vi "Chronos TDMS File Viewer Add Plot.vi"(4 "Data Units":string, 6 "Group":string, 8 "Times":dbl[](array[numeric]), 9 "Data":dbl[](array[numeric]), 10 "Name":string, 11 "Limit Plot Map":T1) -> (3 "Plot Map out":T1)   [LabVIEW 2021]
uses:
  GUI/Chronos cluster Map Limit Plots.ctl
  typedefs/Chronos cluster Plot Data and Limits.ctl
  cluster CC Channel from TDMS.ctl
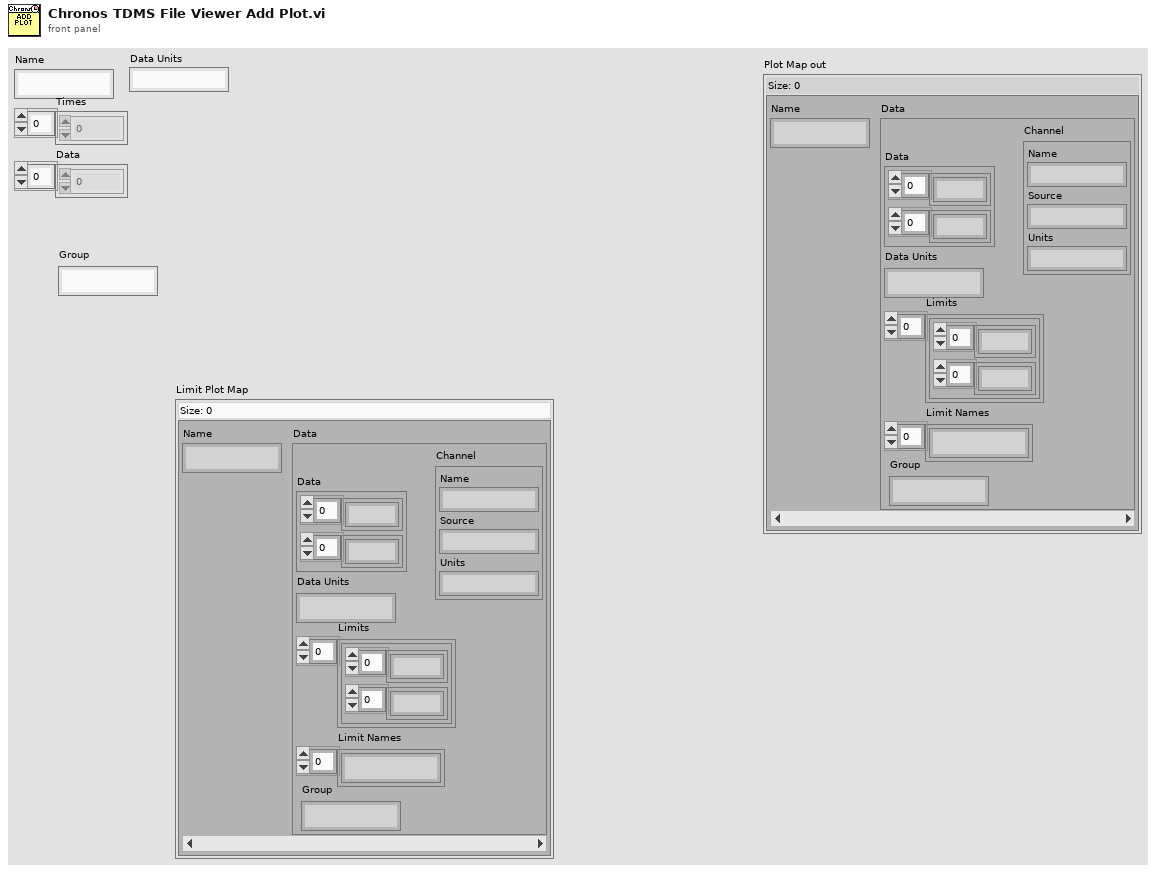
[diagram p1: front panel]
types:
  T1 = typedef "Chronos cluster Map Limit Plots.ctl" = map{string, T2}
  T2 = typedef "Chronos cluster Plot Data and Limits.ctl" = cluster{"Data":cluster{dbl[], dbl[]}, "Data Units":string, "Limits":cluster{dbl[], dbl[]}[], "Limit Names":string[], "Channel":T3, "Group":string}
  T3 = typedef "cluster CC Channel from TDMS.ctl" = cluster{"Name":string, "Source":string, "Units":string}
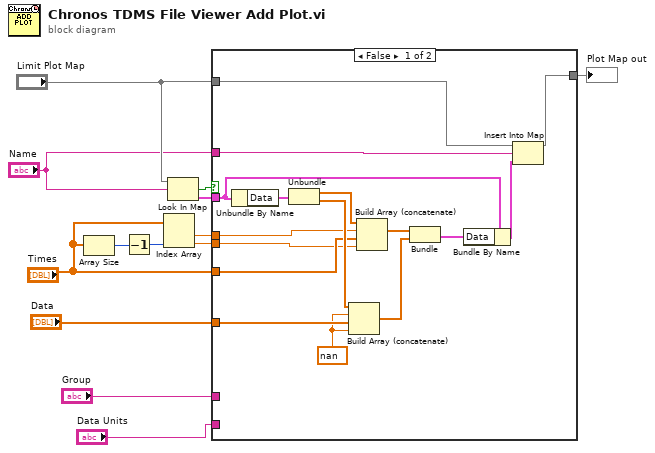
[diagram p0: block diagram]
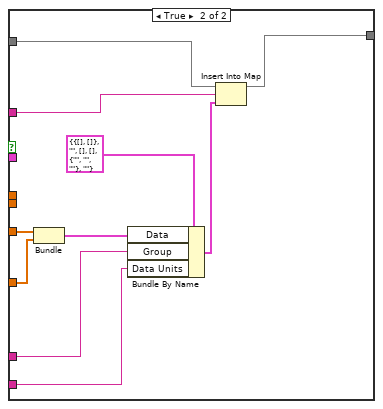
[diagram p2: hidden frame]
diagram:
  n1 = Array Size(array="Times") -> (size(s)=w4:i32)
  n2 = Decrement(x=w4) -> (x-1=w5:i32)
  n3 = Index Array(array="Times", index #2=w5) -> (element #1=w7:dbl, element #2=w3:dbl)  [unwired: 1 in]
  n4 = Look In Map(map="Limit Plot Map", key="Name") -> (key not found?=w13:bool, value=w12:T2)  [unwired: 1 in]
  n5 = case shown="False" w13 {
    tunnel: "Times" -> [w23 w38]
    tunnel: "Data" -> [w28 w39]
    tunnel: w12 -> [w20 _]
    tunnel: "Limit Plot Map" -> [w21 w37]
    tunnel: "Name" -> [w18 w36]
    tunnel: [w17 w34] -> w9
    tunnel: w7 -> [w16 _]
    tunnel: w3 -> [w15 _]
    tunnel: "Group" -> [_ w31]
    tunnel: "Data Units" -> [_ w30]
    frame False {
      w26 = nan
      n6 = Unbundle By Name(w20) -> ("Data"=w22:cluster{dbl[], dbl[]})
      n7 = Unbundle(w22) -> (w29:dbl[], w27:dbl[])
      n8 = Build Array (concatenate)(w27, w26, w28, w26) -> (w24:dbl[])
      n9 = Build Array (concatenate)(w29, w16, w23, w15) -> (w25:dbl[])
      n10 = Bundle(w25, w24) -> (w14:cluster{dbl[], dbl[]})  [unwired: 1 in]
      n11 = Bundle By Name(cluster=w20, "Data"=w14) -> (w19:T2)
      n12 = Insert Into Map(map in=w21, key=w18, value=w19) -> (map out=w17:T1)  [unwired: 2 out]
    }
    frame True {
      n13 = Bundle("Times"=w38, "Data"=w39) -> (w35:cluster{"Times":dbl[], "Data":dbl[]})  [unwired: 1 in]
      n14 = Bundle By Name(cluster=T2 {"Data"={[], []}, "Data Units"="", "Limits"=[], "Limit Names"=[], "Channel"={"Name"="", "Source"="", "Units"=""}, "Group"=""} ("value"), "Data"=w35, "Group"=w31, "Data Units"=w30) -> (w32:T2)
      n15 = Insert Into Map(map in=w37, key=w36, value=w32) -> (map out=w34:T1)  [unwired: 2 out]
    }
  }
  "Plot Map out" <- w9
